vi "SysLogHistory Datei lesen cRIO.vi"(7 "History File":string, 8 "Fehler (in)":errorcluster caption="Fehlerkonstante") -> (0 "Fehler (out)":errorcluster caption="Fehlerkonstante", 3 "Array-Typ (2D Dbl)":string[][](array[string]))   [LabVIEW 2015, in "SysLog.lvlib"]
uses:
  SysLog.lvlib
  <vilib>/WebDAVClient/Simple Get Buffer.vi
  <vilib>/FTP/NI_FTP.lvlib
  <vilib>/WebDAVClient/NI_WebDAV.lvlib
panel:
  out "file error":errorcluster
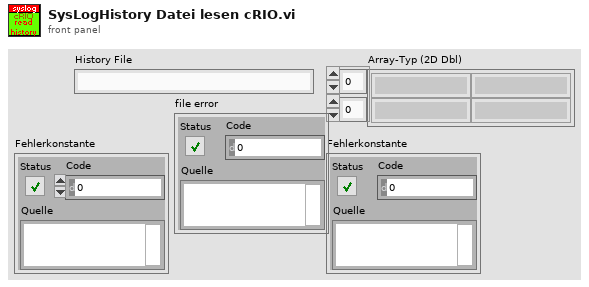
[diagram p1: front panel]
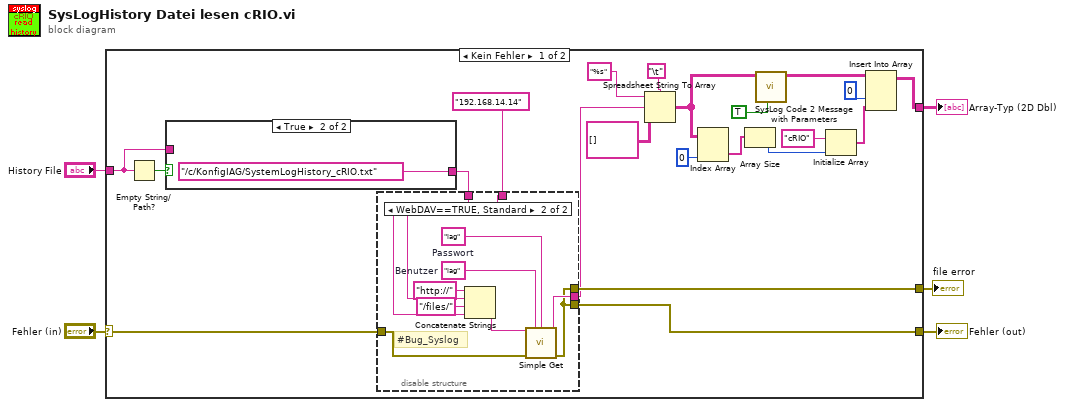
[diagram p0: block diagram]
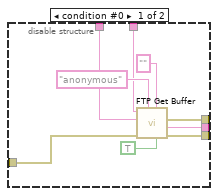
[diagram p2: hidden frame]
diagram:
  n1 = case shown="Kein Fehler" "Fehler (in)" {
    selector: "Fehler (in)" -> [w17 w48]
    tunnel: [w16 w48] -> w4
    tunnel: [w25 _] -> w3
    tunnel: "History File" -> [w18 _]
    tunnel: [w14 _] -> w1
    frame No Error {
      n2 = Empty String/Path?(string/path=w18) -> (empty?=w19:bool)
      n3 = case shown="True" w19 {
        tunnel: w18 -> [w46 _]
        tunnel: [w46 "/c/KonfigIAG/SystemLogHistory_cRIO.txt"] -> w15
        frame False {
        }
        frame True {
        }
      }
      n4 = disable-structure shown="WebDAV==TRUE, Standard" {
        disable-tunnel: w17 -> [w35 w38]
        disable-tunnel: [w34 w36] -> w16
        disable-tunnel: w15 -> [w33 w42]
        disable-tunnel: [w30 w36] -> w14
        disable-tunnel: [w28 w37] -> w13
        disable-tunnel: "192.168.14.14" -> [w27 w43]
        frame condition #0 {
          n5 = call <vilib>:"FTP Get Buffer.vi"("active (T)"=TRUE, "password"="", "user"="anonymous", "error in (no error)"=w35, "remote path"=w33, "host"=w27) -> ("error out"=w34:errorcluster, "data"=w28:string, "file error"=w30:errorcluster)  [unwired: 3 in]
        }
        frame condition #1 (active) {
          w41 = "iag"  # Passwort
          w40 = "iag"  # Benutzer
          # "#Bug_Syslog"
          n6 = Concatenate Strings("http://" ("String"), w43, "/files/" ("String"), w42) -> (w39:string)
          n7 = call-poly <vilib>:"Simple Get.vi"("remote file uri"=w39, "username"=w40, "password"=w41, "error in (no error)"=w38) -> ("data"=w37:string, "error out"=w36:errorcluster)  [unwired: 10 in]
        }
      }
      n8 = Spreadsheet String To Array(delimiter (Tab)="\t", format string="%s" ("Tabellen-String"), spreadsheet string=w13, array type (2D Dbl)=string[][] [] ("Array-Typ (2D Dbl)")) -> (array=w8:string[][])
      n9 = Index Array(array=w8, index (col)=0 ("Deaktivierter Index (Spalte)")) -> (element=w21:string[])  [unwired: 1 in]
      n10 = Array Size(array=w21) -> (size(s)=w20:i32)
      n11 = call "SysLog Code 2 Message with Parameters.vi"("cRIO"=TRUE, "Array-Typ (2D Dbl) (Eingang)"=w8) -> ("Array-Typ (2D Dbl) (Ausgang)"=w7:string[][])  [unwired: 9 in]
      n12 = Initialize Array("cRIO", w20) -> (w23:string[])
      n13 = Insert Into Array(array=w7, index (col)=0 ("Index (Zeile)"), new element=w23) -> (w25:string[][])  [unwired: 1 in]
    }
    frame Error {
    }
  }
  "Fehler (out)" <- w4
  "Array-Typ (2D Dbl)" <- w3
  "file error" <- w1
